vi "SIMPID(v.2).vi"(3 "Range":dbl=10.0, 5 "upper limit":dbl=1.0, 7 "lower limit":dbl=0.4, 9 "Current Point":dbl(knob) scale=0.0..200.0, 10 "Set Point":dbl(knob) scale=0.0..200.0) -> (0 "On Target":bool, 1 "result":dbl)   [LabVIEW 2011]
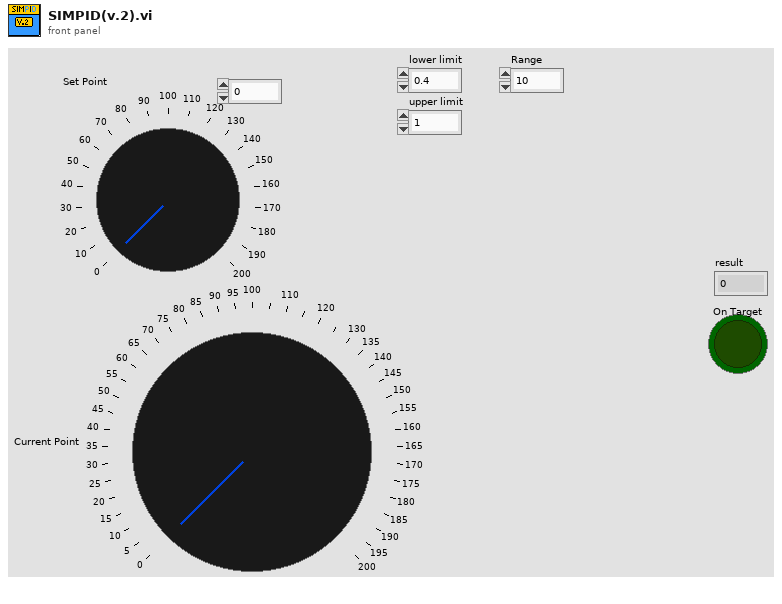
[diagram p1: front panel]
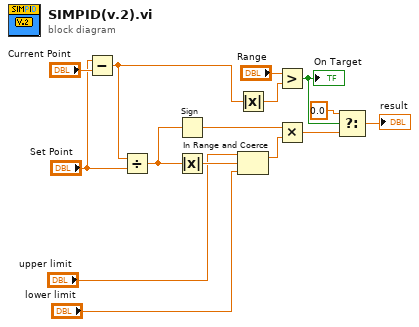
[diagram p0: block diagram]
diagram:
  n1 = Subtract(x="Set Point", y="Current Point") -> (x-y=w2:dbl)
  n2 = Divide(x=w2, y="Set Point") -> (x/y=w12:dbl)
  n3 = Sign(1:w12) -> (0:w9:dbl)
  n4 = Absolute Value(x=w12) -> (abs(x)=w13:dbl)
  n5 = Absolute Value(x=w2) -> (abs(x)=w7:dbl)
  n6 = In Range and Coerce(upper limit="upper limit", x=w13, lower limit="lower limit") -> (coerced(x)=w8:dbl)  [unwired: 1 out]
  n7 = Greater?(x="Range", y=w7) -> (0:w6:bool)
  "On Target" <- w6
  n8 = Multiply(x=w9, y=w8) -> (x*y=w1:dbl)
  n9 = Select(t=0.0, s=w6, f=w1) -> (s? t:f=→"result":dbl)
